vi "MEF_DATA_DYN.vi"(8 "errin":errorcluster, 10 "pathin":path, 11 "datain":T1) -> (0 "error out":errorcluster, 2 "Chaîne":string, 3 "résultat":bool)   [LabVIEW 2020]
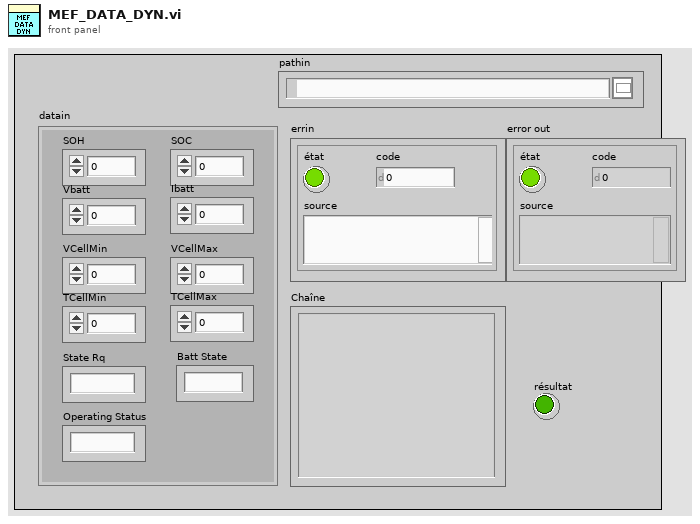
[diagram p1: front panel]
types:
  T1 = cluster{"SOH":dbl, "SOC":dbl, "Vbatt":u32, "Ibatt":dbl, "VCellMax":u32, "VCellMin":u32, "TCellMin":i32, "TCellMax":i32, "State Rq":string, "Batt State":string, "Operating Status":string}
  T2 = cluster{"SOH":dbl, "SOCmin":dbl, "SOCmax":dbl, "Tcellminmin":dbl, "Tcellmaxmax":dbl, "StateRq":string, "BattState":string, "OpStatus":string, "Vcellminmin":dbl, "Vcellmaxmax":dbl, "Vbattmax":dbl, "Vbattmin":dbl}
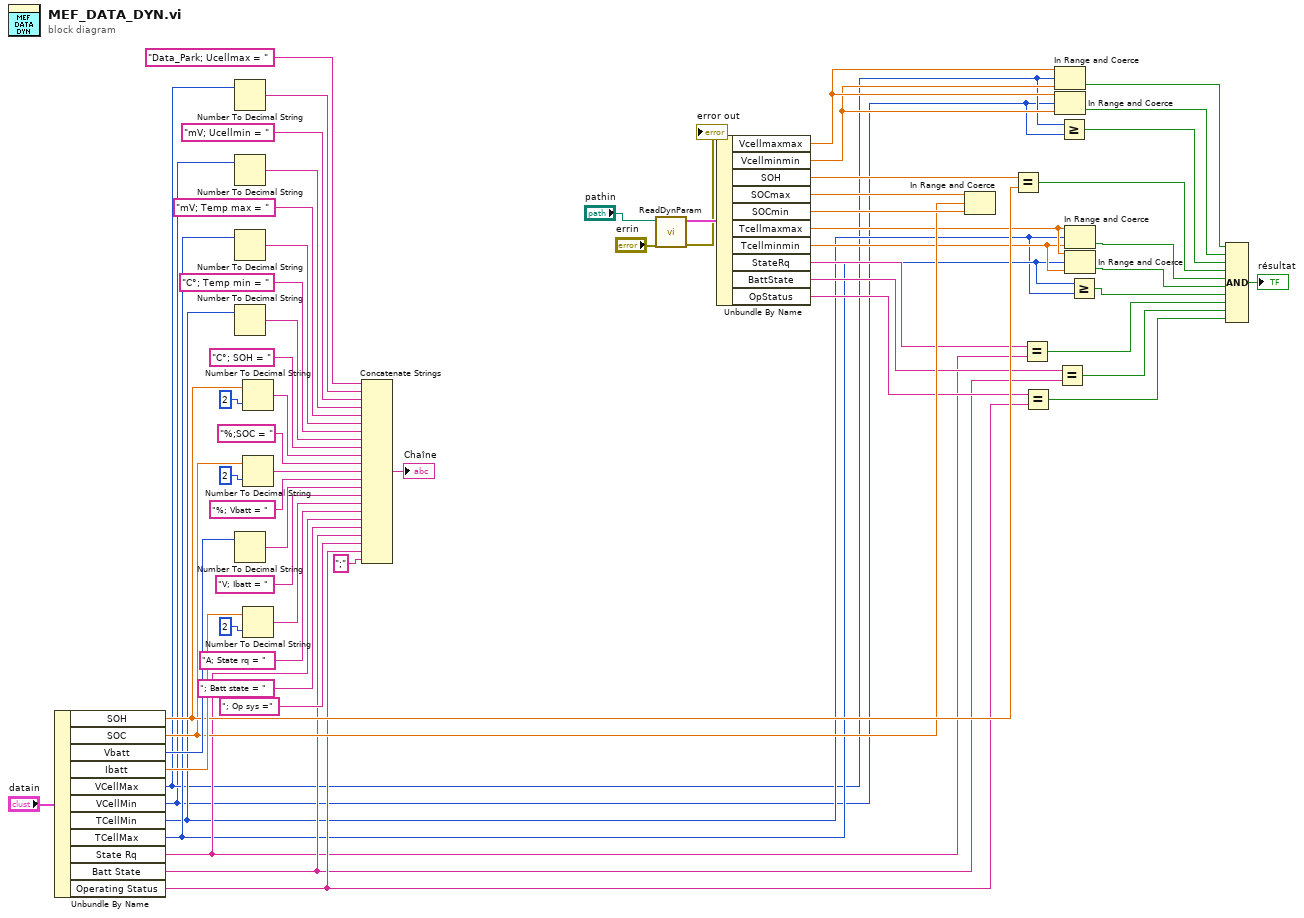
[diagram p0: block diagram]
diagram:
  n1 = Unbundle By Name("datain") -> ("SOH"=w30:dbl, "SOC"=w27:dbl, "Vbatt"=w45:u32, "Ibatt"=w42:dbl, "VCellMax"=w14:u32, "VCellMin"=w13:u32, "TCellMin"=w17:i32, "TCellMax"=w18:i32, "State Rq"=w21:string, "Batt State"=w22:string, "Operating Status"=w23:string)
  n2 = Number To Decimal String(number=w14) -> (decimal integer string=w52:string)  [unwired: 1 in]
  n3 = Number To Decimal String(number=w13) -> (decimal integer string=w53:string)  [unwired: 1 in]
  n4 = Number To Decimal String(number=w18) -> (decimal integer string=w54:string)  [unwired: 1 in]
  n5 = Number To Decimal String(number=w17) -> (decimal integer string=w55:string)  [unwired: 1 in]
  n6 = Number To Decimal String(number=w45) -> (decimal integer string=w46:string)  [unwired: 1 in]
  n7 = Number To Decimal String(number=w30, width (-)=i16 2 ("largeur (-)")) -> (decimal integer string=w56:string)
  n8 = Number To Decimal String(number=w27, width (-)=i16 2 ("largeur (-)")) -> (decimal integer string=w48:string)
  n9 = Number To Decimal String(number=w42, width (-)=i16 2 ("largeur (-)")) -> (decimal integer string=w43:string)
  n10 = Concatenate Strings("Data_Park; Ucellmax = " ("chaîne"), w52, "mV; Ucellmin = " ("chaîne"), w53, "mV; Temp max = " ("chaîne"), w54, "C°; Temp min = " ("chaîne"), w55, "C°; SOH = " ("chaîne"), w56, "%;SOC = " ("chaîne"), w48, "%; Vbatt = " ("chaîne"), w46, "V; Ibatt = " ("chaîne"), w43, "A; State rq = " ("chaîne"), w21, "; Batt state = " ("chaîne"), w22, "; Op sys =" ("chaîne"), w23, ";" ("chaîne")) -> (→"Chaîne":string)
  n11 = call "ReadDynParam.vi"("errin"="errin", "pathin"="pathin") -> ("error out"=→"error out":errorcluster, "DATA"=w32:T2)  [unwired: 8 in]
  n12 = Unbundle By Name(w32) -> ("Vcellmaxmax"=w16:dbl, "Vcellminmin"=w15:dbl, "SOH"=w31:dbl, "SOCmax"=w29:dbl, "SOCmin"=w28:dbl, "Tcellmaxmax"=w20:dbl, "Tcellminmin"=w19:dbl, "StateRq"=w26:string, "BattState"=w25:string, "OpStatus"=w24:string)
  n13 = In Range and Coerce(upper limit=w29, x=w27, lower limit=w28) -> ()  [unwired: 2 out]
  n14 = Equal?(x=w31, y=w30) -> (x = y?=w9:bool)
  n15 = Equal?(x=w26, y=w21) -> (x = y?=w5:bool)
  n16 = Equal?(x=w24, y=w23) -> (x = y?=w3:bool)
  n17 = In Range and Coerce(upper limit=w16, x=w14, lower limit=w15) -> (In Range?=w12:bool)  [unwired: 1 out]
  n18 = In Range and Coerce(upper limit=w16, x=w13, lower limit=w15) -> (In Range?=w11:bool)  [unwired: 1 out]
  n19 = Equal?(x=w25, y=w22) -> (x = y?=w4:bool)
  n20 = Greater Or Equal?(x=w14, y=w13) -> (x >= y?=w10:bool)
  n21 = In Range and Coerce(upper limit=w20, x=w17, lower limit=w19) -> (In Range?=w8:bool)  [unwired: 1 out]
  n22 = In Range and Coerce(upper limit=w20, x=w18, lower limit=w19) -> (In Range?=w7:bool)  [unwired: 1 out]
  n23 = Greater Or Equal?(x=w18, y=w17) -> (x >= y?=w6:bool)
  n24 = Compound Arithmetic op=AND ("Opérateur arithmétique")(w12, w11, w10, w9, w8, w7, w6, w5, w4, w3) -> (→"résultat":bool)
